vi "Read_Wrap_Simple.vi"(4 "Numeric in":refnum<class "Var_I64.lvclass">) -> (1 "Value":T1)   [LabVIEW 2021, in "Var_I64.lvclass"]
uses:
  Var_I64.lvclass
  Type.ctl
  Var_I64.lvclass/Var_I64.ctl
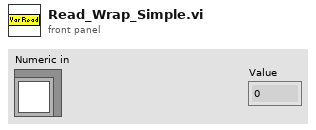
[diagram p1: front panel]
types:
  T1 = typedef "Var_I64.lvclass/Type.ctl" = dbl
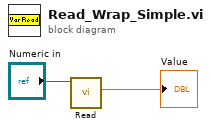
[diagram p0: block diagram]
diagram:
  n1 = call-dynamic "Read.vi"("Numeric in"="Numeric in") -> ("Numeric"=→"Value":T1)  [unwired: 8 in, 2 out]
